vi "Old Files Handler.vi"(8 "Error In":errorcluster, 11 "TDMS Log":refnum<class "TDMS Logger.lvclass">) -> (0 "Error Out":errorcluster, 3 "TDMS Log":refnum<class "TDMS Logger.lvclass">)   [LabVIEW 2014, in "TDMS Logger.lvlib" / "TDMS Logger.lvclass"]
uses:
  TDMS Logger.lvclass
  TDMS Logger.lvclass/TDMS Logger.ctl
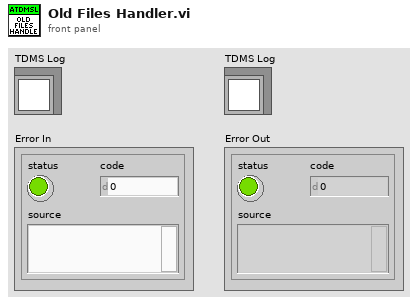
[diagram p1: front panel]
types:
  T1 = typedef "TDMS Logger.lvlib/TDMS Logger.lvclass/Folder Size Limit Reached.ctl" = enum16{"Do Nothing", "Remove Oldest Files"}
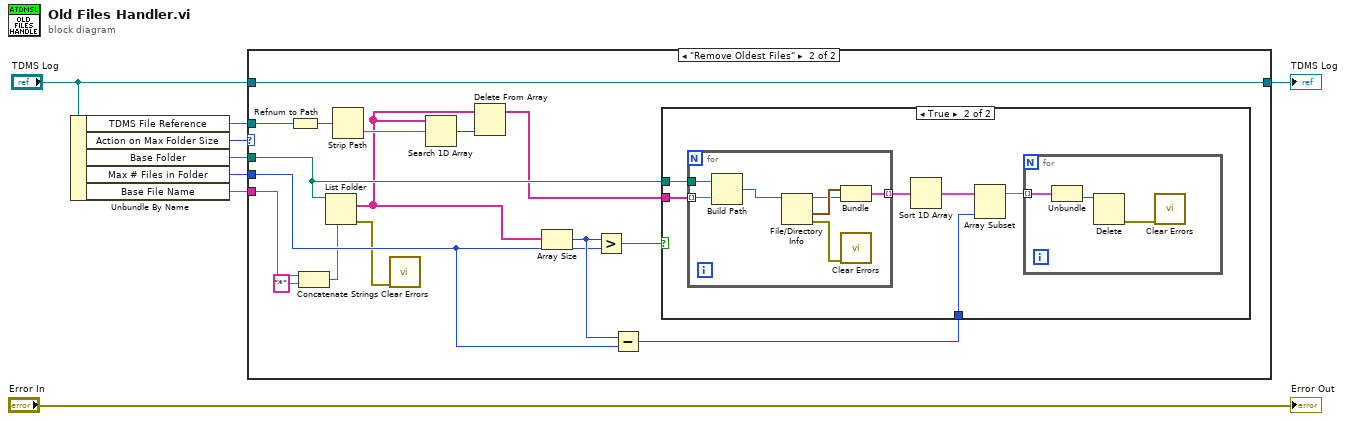
[diagram p0: block diagram]
diagram:
  n1 = Unbundle By Name("TDMS Log") -> ("TDMS File Reference"=w3:refnum<k34>, "Action on Max Folder Size"=w5:T1, "Base Folder"=w4:path, "Max # Files in Folder"=w6:i32, "Base File Name"=w1:string)
  n2 = case shown="\"Remove Oldest Files\"" w5 {
    tunnel: w4 -> [_ w23]
    tunnel: w6 -> [_ w21]
    tunnel: "TDMS Log" -> [w9 w24]
    tunnel: [w9 w24] -> w8
    tunnel: w3 -> [_ w19]
    tunnel: w1 -> [_ w15]
    frame "Do Nothing", Default {
    }
    frame "Remove Oldest Files" {
      n3 = Refnum to Path(1:w19) -> (0:w18:path)
      n4 = Concatenate Strings(w15, "*" ("string")) -> (w14:string)
      n5 = List Folder(path=w23, pattern=w14) -> (filenames=w10:string[], error out=w12:errorcluster)  [unwired: 2 in, 2 out]
      n6 = Strip Path(path=w18) -> (name=w17:string)  [unwired: 1 out]
      n7 = call <vilib>:"Clear Errors.vi"("error in (no error)"=w12) -> ()  [unwired: 5 in, 2 out]
      n8 = Search 1D Array(1D array=w10, element=w17) -> (index of element=w16:i32)  [unwired: 1 in]
      n9 = Delete From Array(array=w10, index=w16) -> (array with subset deleted=w11:string[])  [unwired: 1 in, 1 out]
      n10 = Array Size(array=w10) -> (size(s)=w22:i32)
      n11 = Greater?(x=w22, y=w21) -> (0:w25:bool)
      n12 = Subtract(x=w22, y=w21) -> (x-y=w20:i32)
      n13 = case shown="True" w25 {
        tunnel: w11 -> [_ w31]
        tunnel: w23 -> [_ w27]
        tunnel: w20 -> [_ w26]
        frame False {
        }
        frame True {
          n14 = for {
            tunnel: w31 -> [w38] mode=indexing
            tunnel: [w40] -> w30 mode=indexing
            tunnel: w27 -> [w37]
            n15 = Build Path(base path=w37, name or relative path=w38) -> (appended path=w36:path)
            n16 = File/Directory Info(path=w36) -> (path out=w39:path, last mod=w41:timestamp, error out=w35:errorcluster)  [unwired: 1 in, 4 out]
            n17 = Bundle("last mod"=w41, "path out"=w39) -> (w40:cluster{"last mod":timestamp, "path out":path})  [unwired: 1 in]
            n18 = call <vilib>:"Clear Errors.vi"("error in (no error)"=w35) -> ()  [unwired: 5 in, 2 out]
          }
          n19 = Sort 1D Array(array=w30) -> (sorted array=w28:cluster{"last mod":timestamp, "path out":path}[])
          n20 = Array Subset(array=w28, length=w26) -> (w29:cluster{"last mod":timestamp, "path out":path}[])  [unwired: 1 in]
          n21 = for {
            tunnel: w29 -> [w34] mode=indexing
            n22 = Unbundle(w34) -> ("path out"=w33:path)  [unwired: 1 out]
            n23 = Delete(path (use dialog)=w33) -> (error out=w32:errorcluster)  [unwired: 4 in, 2 out]
            n24 = call <vilib>:"Clear Errors.vi"("error in (no error)"=w32) -> ()  [unwired: 5 in, 2 out]
          }
        }
      }
    }
  }
  "TDMS Log" <- w8
  "Error Out" <- "Error In"
